vi "set up acquisition parameters.vi"(6 "error in (no error)":errorcluster, 7 "Acquisition Parameters":T2={"Readout Mode"=enum."Full Vertical Binning", "Set Acquisition Mode"=enum."(do nothing)", "Trigger Mode"=enum."Internal", "Exposure Time (sec)"=0.0, "Accumulation Cycle (s)"=0.0, "Kinetic Cycle Time (s)"=0.0, "Number of Kinetics"=0, "Number of Accumulations"=0, "Set VS Speed"=0.0, "Pixel Rate"=enum."Standard CCD 3 Mhz 14 bits", "V Shift Amplitude"=enum."+1", "Preamp Gain"=enum."1.0", "Single Track Settings"={"centre"=0, "height"=1}, "EM CCD Gain"=300, "High Capacity?"=FALSE} {"EM CCD Gain" scale=0.01..300.0; "Single Track Settings"."centre" min=0 max=1024; "Single Track Settings"."height" min=1 max=1024; "Exposure Time (sec)" scale=0.001..10.0 scale format="%#_1g"; "Set VS Speed" min=0.0 format="%#_2f"}, 8 "Image Size":T1 {"V Bin" min=0.0; "H Bin" min=0.0 step=1.0}) -> (0 "error out":errorcluster, 1 "Kinetics":dbl format="%#_13g", 2 "Accumulation":dbl format="%#_13g", 3 "Exposure":dbl format="%#_13g")   [LabVIEW 2014]
uses:
  ctt's/Camera Setup Acquisition.ctl
  ctt's/Image size and binning.ctl
  Globals/Initilize Globals.vi
  Library Files - Andor and MadCity/Andorlib/atmcd32d.lvlib
  Library Files - Andor and MadCity/Andorlib/atmcd32d.dll
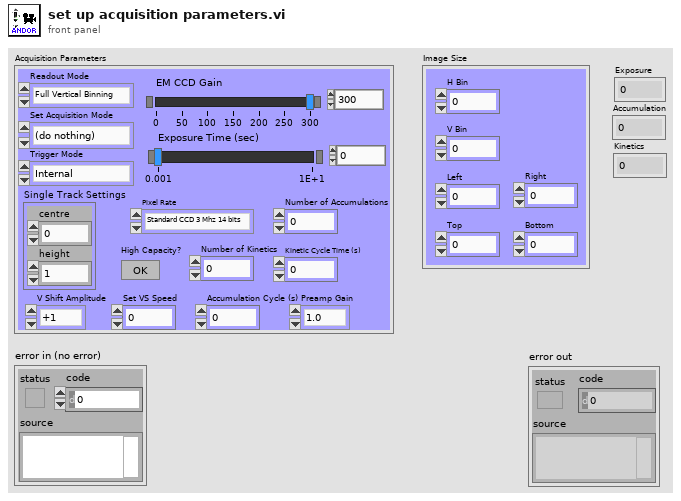
[diagram p1: front panel]
types:
  T1 = typedef "Image size and binning.ctl" = cluster{"H Bin":dbl, "V Bin":dbl, "Left":dbl, "Right":dbl, "Top":dbl, "Bottom":dbl}
  T2 = typedef "Camera Setup Acquisition.ctl" = cluster{"Readout Mode":enum16{"Full Vertical Binning", "Multi-Track", "Random-Track", "Single-Track", "Image"}, "Set Acquisition Mode":enum16{"(do nothing)", "Single Scan", "Accumulate", "Kinetics", "Fast Kinetics", "Run till abort"}, "Trigger Mode":enum16{"Internal", "External"}, "Exposure Time (sec)":sgl, "Accumulation Cycle (s)":dbl, "Kinetic Cycle Time (s)":dbl, "Number of Kinetics":i32, "Number of Accumulations":i32, "Set VS Speed":dbl, "Pixel Rate":enum16{"EM CCD 10 Mhz 14 bits", "EM CCD 5 Mhz 14 bits", "EM CCD 3 Mhz 14 bits", "EM CCD 1 Mhz 16 bits", "Standard CCD 3 Mhz 14 bits", "Standard CCD 1 Mhz 16 bits"}, "V Shift Amplitude":enum16{"normal", "+1", "+2", "+3", "+4"}, "Preamp Gain":enum16{"1.0", "2.4", "5.0"}, "Single Track Settings":cluster{"centre":i32, "height":i32}, "EM CCD Gain":u16, "High Capacity?":bool}
  T3 = enum16{"(do nothing)", "Single Scan", "Accumulate", "Kinetics", "Fast Kinetics", "Run till abort"}
  T4 = cluster{"Adc Channel":i32, "H Shift Setting":i32, "EM on?":bool}[]
  T5 = enum16{"Full Vertical Binning", "Multi-Track", "Random-Track", "Single-Track", "Image"}
  T6 = enum16{"EM CCD 10 Mhz 14 bits", "EM CCD 5 Mhz 14 bits", "EM CCD 3 Mhz 14 bits", "EM CCD 1 Mhz 16 bits", "Standard CCD 3 Mhz 14 bits", "Standard CCD 1 Mhz 16 bits"}
  T7 = cluster{"Adc Channel":i32, "H Shift Setting":i32, "EM on?":bool}
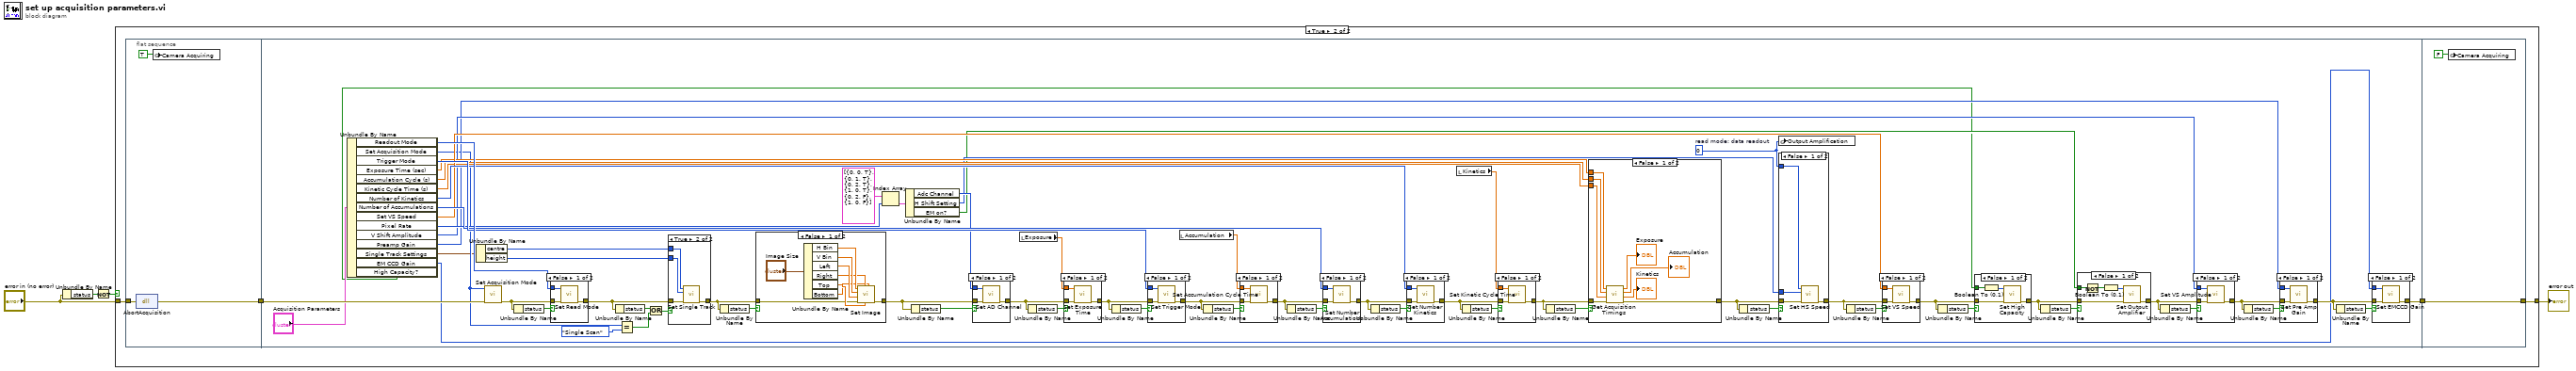
[diagram p0: block diagram]
diagram:
  n1 = Unbundle By Name("error in (no error)") -> ("status"=w4:bool)
  n2 = Not(x=w4) -> (.not. x?=w3:bool)
  n3 = case shown="True" w3 {
    tunnel: "error in (no error)" -> [w5 w8]
    tunnel: [w5 w7] -> w1
    frame False {
    }
    frame True {
      n4 = flat-sequence {
        tunnel: [w11] -> w9
        tunnel: w8 -> [w12]
        tunnel: w9 -> [w28]
        tunnel: [w27] -> w6
        tunnel: [w169] -> w7
        tunnel: w6 -> [w169]
        frame #0 {
          n5 = dll-call lib="C:/Users/Lambda2/Desktop/Testing/Testing-Lambda/TIRF-Microscope/Library Files - Andor and MadCity/Andorlib/ATMCD32D.DLL" fn="AbortAcquisition" label="Call Library Function\nAbort"(error in=w12) -> (error out=w11:errorcluster)  [unwired: 2 in, 2 out]
          n6 = global write "Initilize Globals.vi" "Camera Acquiring"(TRUE) -> ()
        }
        frame #1 {
          w41 = 0  # read mode: data readout
          n7 = Unbundle By Name("Acquisition Parameters") -> ("Readout Mode"=w61:T5, "Set Acquisition Mode"=w24:T3, "Trigger Mode"=w60:enum16{"Internal", "External"}, "Exposure Time (sec)"=w55:sgl, "Accumulation Cycle (s)"=w56:dbl, "Kinetic Cycle Time (s)"=w54:dbl, "Number of Kinetics"=w58:i32, "Number of Accumulations"=w59:i32, "Set VS Speed"=w57:dbl, "Pixel Rate"=w48:T6, "V Shift Amplitude"=w30:enum16{"normal", "+1", "+2", "+3", "+4"}, "Preamp Gain"=w29:enum16{"1.0", "2.4", "5.0"}, "Single Track Settings"=w17:cluster{"centre":i32, "height":i32}, "EM CCD Gain"=w14:u16, "High Capacity?"=w13:bool)
          n8 = Unbundle By Name(w17) -> ("centre"=w16:i32, "height"=w15:i32)
          n9 = call "Set Acquisition Mode.vi"("error in (no error)"=w28, "mode"=w24) -> ("error out"=w63:errorcluster)  [unwired: 8 in, 1 out]
          n10 = Unbundle By Name(w63) -> ("status"=w64:bool)
          n11 = case shown="False" w64 {
            tunnel: w63 -> [w125 w126]
            tunnel: [w124 w126] -> w21
            tunnel: w61 -> [w123 _]
            frame False {
              n12 = call "Set Read Mode.vi"("error in (no error)"=w125, "mode"=w123) -> ("error out"=w124:errorcluster)  [unwired: 8 in, 1 out]
            }
            frame True {
            }
          }
          n13 = Unbundle By Name(w21) -> ("status"=w19:bool)
          n14 = Equal?(x=w24, y=T3."Single Scan") -> (x = y?=w20:bool)
          n15 = Or(x=w19, y=w20) -> (x .or. y?=w18:bool)
          n16 = case shown="True" w18 {
            tunnel: w21 -> [w81 w85]
            tunnel: [w81 w84] -> w22
            tunnel: w16 -> [_ w83]
            tunnel: w15 -> [_ w82]
            frame False {
            }
            frame True {
              n17 = call "Set Single Track.vi"("error in (no error)"=w85, "height"=w82, "centre"=w83) -> ("error out"=w84:errorcluster)  [unwired: 7 in, 1 out]
            }
          }
          n18 = Unbundle By Name(w22) -> ("status"=w50:bool)
          n19 = case shown="False" w50 {
            tunnel: w22 -> [w114 w122]
            tunnel: [w113 w122] -> w44
            frame False {
              n20 = Unbundle By Name("Image Size") -> ("H Bin"=w120:dbl, "V Bin"=w119:dbl, "Left"=w118:dbl, "Right"=w117:dbl, "Top"=w116:dbl, "Bottom"=w115:dbl)
              n21 = call "Set Image.vi"("vend"=w115, "vstart"=w116, "hend"=w117, "error in (no error)"=w114, "hstart"=w118, "vbin"=w119, "hbin"=w120) -> ("error out"=w113:errorcluster)  [unwired: 3 in, 1 out]
            }
            frame True {
            }
          }
          n22 = Index Array(array=T4 [{"Adc Channel"=0, "H Shift Setting"=0, "EM on?"=TRUE}, {"Adc Channel"=0, "H Shift Setting"=1, "EM on?"=TRUE}, {"Adc Channel"=0, "H Shift Setting"=2, "EM on?"=TRUE}, {"Adc Channel"=1, "H Shift Setting"=0, "EM on?"=TRUE}, {"Adc Channel"=0, "H Shift Setting"=2, "EM on?"=FALSE}, {"Adc Channel"=1, "H Shift Setting"=0, "EM on?"=FALSE}], index=w48) -> (element=w47:T7)
          n23 = Unbundle By Name(w47) -> ("Adc Channel"=w43:i32, "H Shift Setting"=w42:i32, "EM on?"=w31:bool)
          n24 = Unbundle By Name(w44) -> ("status"=w46:bool)
          n25 = case shown="False" w46 {
            tunnel: [w110 w112] -> w45
            tunnel: w44 -> [w111 w112]
            tunnel: w43 -> [w109 _]
            frame False {
              n26 = call "Set AD Channel.vi"("error in (no error)"=w111, "channel"=w109) -> ("error out"=w110:errorcluster)  [unwired: 8 in, 1 out]
            }
            frame True {
            }
          }
          n27 = local read "Exposure"() -> (w53:dbl)
          n28 = Unbundle By Name(w45) -> ("status"=w62:bool)
          n29 = case shown="False" w62 {
            tunnel: w45 -> [w167 w168]
            tunnel: [w166 w168] -> w72
            tunnel: w53 -> [w165 _]
            frame False {
              n30 = call "Set Exposure Time.vi"("error in (no error)"=w167, "time"=w165) -> ("error out"=w166:errorcluster)  [unwired: 8 in, 1 out]
            }
            frame True {
            }
          }
          n31 = Unbundle By Name(w72) -> ("status"=w80:bool)
          n32 = case shown="False" w80 {
            tunnel: w72 -> [w163 w164]
            tunnel: [w162 w164] -> w71
            tunnel: w60 -> [w161 _]
            frame False {
              n33 = call "Set Trigger Mode.vi"("error in (no error)"=w163, "mode"=w161) -> ("error out"=w162:errorcluster)  [unwired: 8 in, 1 out]
            }
            frame True {
            }
          }
          n34 = local read "Accumulation"() -> (w52:dbl)
          n35 = Unbundle By Name(w71) -> ("status"=w79:bool)
          n36 = case shown="False" w79 {
            tunnel: w71 -> [w159 w160]
            tunnel: [w158 w160] -> w70
            tunnel: w52 -> [w157 _]
            frame False {
              n37 = call "Set Accumulation Cycle Time.vi"("error in (no error)"=w159, "time"=w157) -> ("error out"=w158:errorcluster)  [unwired: 8 in, 1 out]
            }
            frame True {
            }
          }
          n38 = Unbundle By Name(w70) -> ("status"=w78:bool)
          n39 = case shown="False" w78 {
            tunnel: w70 -> [w155 w156]
            tunnel: [w154 w156] -> w69
            tunnel: w59 -> [w153 _]
            frame False {
              n40 = call "Set Number Accumulations.vi"("error in (no error)"=w155, "number"=w153) -> ("error out"=w154:errorcluster)  [unwired: 8 in, 1 out]
            }
            frame True {
            }
          }
          n41 = Unbundle By Name(w69) -> ("status"=w77:bool)
          n42 = case shown="False" w77 {
            tunnel: w69 -> [w151 w152]
            tunnel: [w150 w152] -> w68
            tunnel: w58 -> [w149 _]
            frame False {
              n43 = call "Set Number Kinetics.vi"("error in (no error)"=w151, "number"=w149) -> ("error out"=w150:errorcluster)  [unwired: 8 in, 1 out]
            }
            frame True {
            }
          }
          n44 = local read "Kinetics"() -> (w51:dbl)
          n45 = Unbundle By Name(w68) -> ("status"=w76:bool)
          n46 = case shown="False" w76 {
            tunnel: w68 -> [w147 w148]
            tunnel: [w146 w148] -> w67
            tunnel: w51 -> [w145 _]
            frame False {
              n47 = call "Set Kinetic Cycle Time.vi"("error in (no error)"=w147, "time"=w145) -> ("error out"=w146:errorcluster)  [unwired: 8 in, 1 out]
            }
            frame True {
            }
          }
          n48 = Unbundle By Name(w67) -> ("status"=w75:bool)
          n49 = case shown="False" w75 {
            tunnel: w67 -> [w143 w144]
            tunnel: [w142 w144] -> w66
            tunnel: w56 -> [w141 _]
            tunnel: w55 -> [w140 _]
            tunnel: w54 -> [w139 _]
            frame False {
              n50 = call "Get Acquisition Timings.vi"("error in (no error)"=w143, "kinetic"=w139, "accumulate"=w141, "exposure"=w140) -> ("error out"=w142:errorcluster, "kinetic out"=→"Kinetics":sgl, "accumulate out"=→"Accumulation":sgl, "exposure out"=→"Exposure":sgl)  [unwired: 3 in, 1 out]
            }
            frame True {
            }
          }
          n51 = Unbundle By Name(w66) -> ("status"=w74:bool)
          n52 = global write "Initilize Globals.vi" "Output Amplification"(w41) -> ()
          n53 = case shown="False" w74 {
            tunnel: w66 -> [w134 w135]
            tunnel: [w133 w135] -> w65
            tunnel: w42 -> [w132 _]
            tunnel: w41 -> [w131 _]
            frame False {
              n54 = call "Set HS Speed.vi"("error in (no error)"=w134, "index"=w132, "typ"=w131) -> ("error out"=w133:errorcluster)  [unwired: 7 in, 1 out]
            }
            frame True {
            }
          }
          n55 = Unbundle By Name(w65) -> ("status"=w73:bool)
          n56 = case shown="False" w73 {
            tunnel: w65 -> [w129 w130]
            tunnel: [w128 w130] -> w35
            tunnel: w57 -> [w127 _]
            frame False {
              n57 = call "Set VS Speed.vi"("error in (no error)"=w129, "index"=w127) -> ("error out"=w128:errorcluster)  [unwired: 8 in, 1 out]
            }
            frame True {
            }
          }
          n58 = Unbundle By Name(w35) -> ("status"=w40:bool)
          n59 = case shown="False" w40 {
            tunnel: [w106 w108] -> w34
            tunnel: w35 -> [w107 w108]
            tunnel: w13 -> [w104 _]
            frame False {
              n60 = Boolean To (0,1)(Boolean=w104) -> (0, 1=w105:i16)
              n61 = call "Set High Capacity.vi"("error in (no error)"=w107, "state"=w105) -> ("error out"=w106:errorcluster)  [unwired: 8 in, 1 out]
            }
            frame True {
            }
          }
          n62 = Unbundle By Name(w34) -> ("status"=w39:bool)
          n63 = case shown="False" w39 {
            tunnel: [w101 w103] -> w33
            tunnel: w34 -> [w102 w103]
            tunnel: w31 -> [w98 _]
            frame False {
              n64 = Not(x=w98) -> (.not. x?=w99:bool)
              n65 = Boolean To (0,1)(Boolean=w99) -> (0, 1=w100:i16)
              n66 = call "Set Output Amplifier.vi"("error in (no error)"=w102, "typ"=w100) -> ("error out"=w101:errorcluster)  [unwired: 8 in, 1 out]
            }
            frame True {
            }
          }
          n67 = Unbundle By Name(w33) -> ("status"=w38:bool)
          n68 = case shown="False" w38 {
            tunnel: [w95 w97] -> w32
            tunnel: w33 -> [w96 w97]
            tunnel: w30 -> [w94 _]
            frame False {
              n69 = call "Set VS Amplitude.vi"("error in (no error)"=w96, "index"=w94) -> ("error out"=w95:errorcluster)  [unwired: 8 in, 1 out]
            }
            frame True {
            }
          }
          n70 = Unbundle By Name(w32) -> ("status"=w37:bool)
          n71 = case shown="False" w37 {
            tunnel: [w91 w93] -> w25
            tunnel: w32 -> [w92 w93]
            tunnel: w29 -> [w90 _]
            frame False {
              n72 = call "Set Pre Amp Gain.vi"("error in (no error)"=w92, "index"=w90) -> ("error out"=w91:errorcluster)  [unwired: 8 in, 1 out]
            }
            frame True {
            }
          }
          n73 = Unbundle By Name(w25) -> ("status"=w36:bool)
          n74 = case shown="False" w36 {
            tunnel: [w87 w89] -> w27
            tunnel: w25 -> [w88 w89]
            tunnel: w14 -> [w86 _]
            frame False {
              n75 = call "Set EMCCD Gain.vi"("error in (no error)"=w88, "gain"=w86) -> ("error out"=w87:errorcluster)  [unwired: 8 in, 1 out]
            }
            frame True {
            }
          }
        }
        frame #2 {
          n76 = global write "Initilize Globals.vi" "Camera Acquiring"(FALSE) -> ()
        }
      }
    }
  }
  "error out" <- w1
